vi "SVM Cross-Validate EPSILON_SVR.vi"(6 "Nr fold":i32 caption="Nr fold (LOO)", 7 "Options":T6={"cache_size"=200.0, "eps"=0.001, "shrinking"=TRUE, "probability"=FALSE}, 8 "error in (no error)":errorcluster, 9 "Param EPSILON_SVR":T1={"C"=1.0, "p"=0.1}, 10 "Kernel":T4, 11 "Problem":T2) -> (0 "error out":errorcluster, 3 "Target":dbl[](array[numeric]) caption="Target (Predicted labels)")   [LabVIEW 2015]
doc: "This function conducts cross validation. Data are separated to nr_fold folds. Under given parameters sequentially each fold is validated using the model from training the remaining. Predicted labels (of all prob's instances) in the validation process are stored in the array called target.\n\nThe default number of folds uses Leave-One-Out cross-validation (LOO)."
uses:
  Controls/Options Training.ctl
  Controls/Kernel.ctl
  Wrapper API/Controls/svm_kernel_type.ctl
  Wrapper API/Controls/svm_problem.ctl
  Wrapper API/Controls/svm_node.ctl
  Controls/Parameters EPSILON_SVR.ctl
  Wrapper API/Controls/svm_parameter.ctl
  Wrapper API/Controls/svm_type.ctl
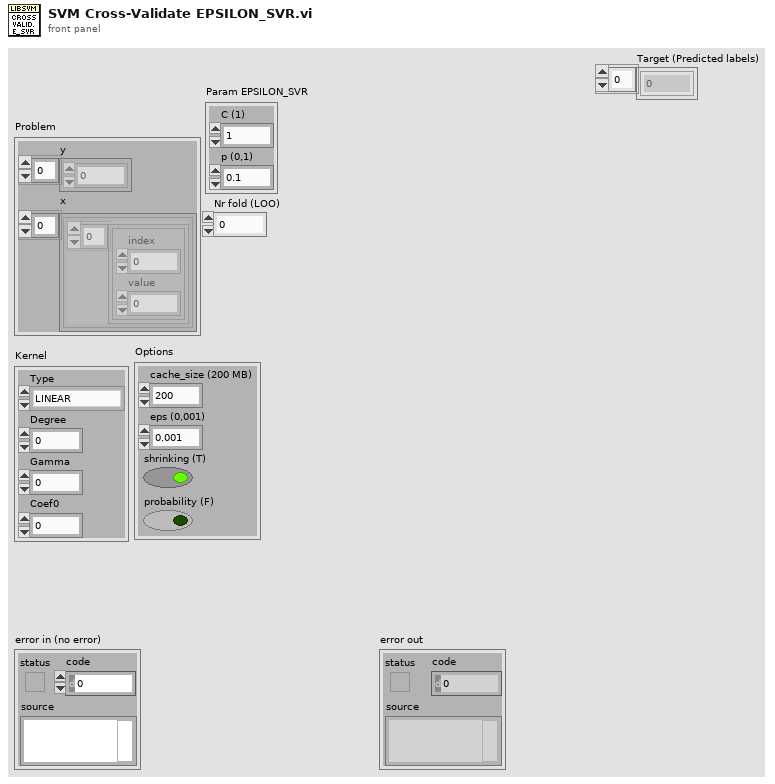
[diagram p1: front panel]
types:
  T1 = typedef "Parameters EPSILON_SVR.ctl" = cluster{"C":dbl, "p":dbl}
  T2 = typedef "svm_problem.ctl" = cluster{"y":dbl[], "x":cluster{T3[]}[]}
  T3 = typedef "svm_node.ctl" = cluster{"index":i32, "value":dbl}
  T4 = typedef "Kernel.ctl" = cluster{"Type":T5, "Degree":i32, "Gamma":dbl, "Coef0":dbl}
  T5 = typedef "svm_kernel_type.ctl" = enum32{"LINEAR", "POLY", "RBF", "SIGMOID", "PRECOMPUTED"}
  T6 = typedef "Options Training.ctl" = cluster{"cache_size":dbl, "eps":dbl, "shrinking":bool, "probability":bool}
  T7 = typedef "svm_type.ctl" = enum32{"C_SVC", "NU_SVC", "ONE_CLASS", "EPSILON_SVR", "NU_SVR"}
  T8 = typedef "svm_parameter.ctl" = cluster{"svm_type":T7, "kernel_type":T5, "degree":i32, "gamma":dbl, "coef0":dbl, "cache_size":dbl, "eps":dbl, "C":dbl, "weight_label":i32[], "weight":dbl[], "nu":dbl, "p":dbl, "shrinking":bool, "probability":bool}
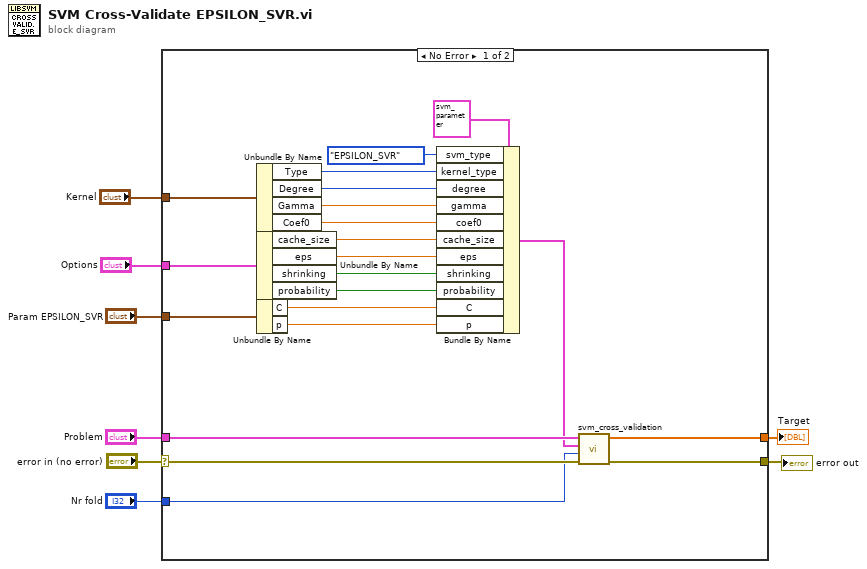
[diagram p0: block diagram]
diagram:
  n1 = case shown="No Error" "error in (no error)" {
    selector: "error in (no error)" -> [w10 w30]
    tunnel: [w11 w30] -> w8
    tunnel: "Problem" -> [w14 _]
    tunnel: "Kernel" -> [w28 _]
    tunnel: [w12 _] -> w1
    tunnel: "Options" -> [w19 _]
    tunnel: "Param EPSILON_SVR" -> [w20 _]
    tunnel: "Nr fold" -> [w9 _]
    frame No Error {
      n2 = Unbundle By Name(w28) -> ("Type"=w27:T5, "Degree"=w26:i32, "Gamma"=w25:dbl, "Coef0"=w24:dbl)
      n3 = Unbundle By Name(w19) -> ("cache_size"=w22:dbl, "eps"=w21:dbl, "shrinking"=w18:bool, "probability"=w17:bool)
      n4 = Unbundle By Name(w20) -> ("C"=w16:dbl, "p"=w15:dbl)
      n5 = Bundle By Name(cluster=T8 {"svm_type"=enum."C_SVC", "kernel_type"=enum."LINEAR", "degree"=0, "gamma"=0.0, "coef0"=0.0, "cache_size"=0.0, "eps"=0.0, "C"=0.0, "weight_label"=[], "weight"=[], "nu"=0.0, "p"=0.0, "shrinking"=FALSE, "probability"=FALSE} ("svm_parameter"), "svm_type"=svm_type."EPSILON_SVR", "kernel_type"=w27, "degree"=w26, "gamma"=w25, "coef0"=w24, "cache_size"=w22, "eps"=w21, "shrinking"=w18, "probability"=w17, "C"=w16, "p"=w15) -> (w13:T8)
      n6 = call "svm_cross_validation.vi"("error in (no error)"=w10, "Nr fold"=w9, "Parameters"=w13, "Problem"=w14) -> ("error out"=w11:errorcluster, "Target"=w12:dbl[])  [unwired: 6 in]
    }
    frame Error {
    }
  }
  "error out" <- w8
  "Target" <- w1
